vi "Connect.vi"(8 "error in (no error)":errorcluster, 9 "timeout_ms (-1)":i32=-1, 11 "INetworkWriter in":refnum<class "INetworkWriter.lvclass">) -> (0 "error out":errorcluster, 3 "INetworkWriter out":refnum<class "INetworkWriter.lvclass">)   [LabVIEW 2024, in "INetworkWriter.lvclass"]
uses:
  INetworkWriter.lvclass
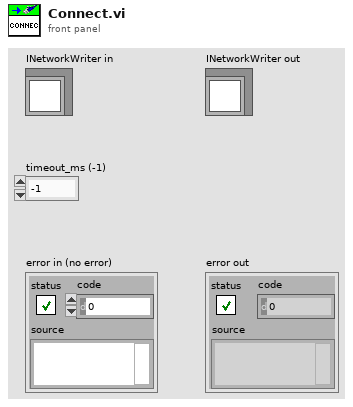
[diagram p1: front panel]
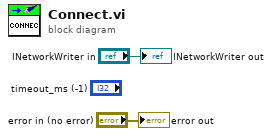
[diagram p0: block diagram]
diagram:
  "error out" <- "error in (no error)"
  "INetworkWriter out" <- "INetworkWriter in"
